vi "ClimbLogic.vi"(0 "FrontClimbEncoder":dbl, 5 "BackClimbEncoder":dbl) -> (4 "ClimbDrive":dbl, 6 "ActuateFrontClimb":dbl, 8 "ActuateBackClimb":dbl)   [LabVIEW 2018]
uses:
  <vilib>/Rock Robotics/WPI/Utilities/WPI_GetSetVariantRefNum.vi
  Swerve/SwerveGlobals.vi
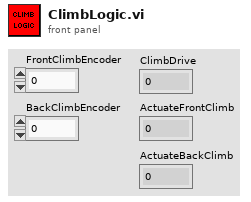
[diagram p1: front panel]
types:
  T1 = typedef "WPI_CompressorDevRef.ctl" = cluster{"DevStatus":errorcluster, "Pneumatics Control Module":u8}
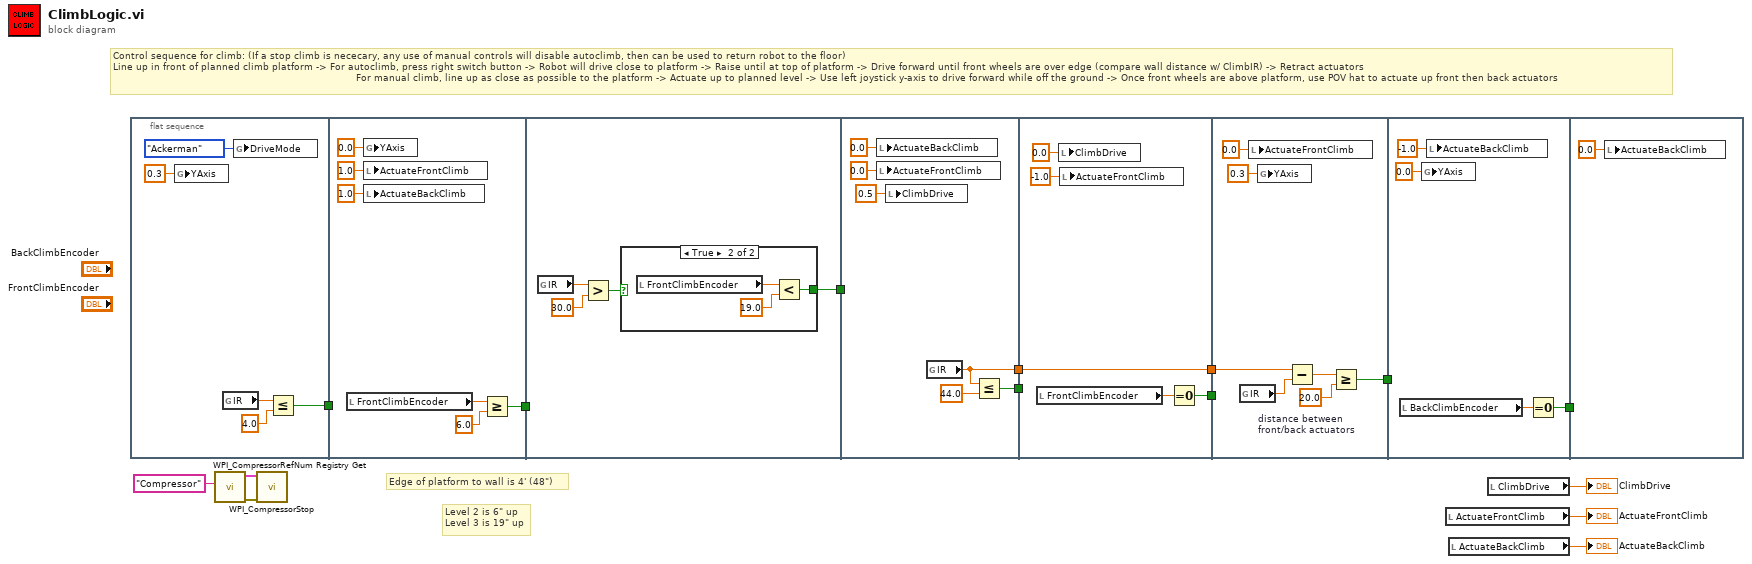
[diagram p0: block diagram]
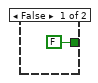
[diagram p2: hidden frame]
diagram:
  # "Level 2 is 6\" up\nLevel 3 is 19\" up"
  # "Edge of platform to wall is 4' (48\")"
  # "Control sequence for climb: (If a stop climb is nececary, any use of manual controls will disable autoclimb, then can be used to return robot to the floor)\nLine up in front of planned climb platform -> For autoclimb, press right switch button -> Robot will drive close to platform -> Raise until at top of platform -> Drive forward until front wheels are over edge (compare wall distance w/ ClimbIR) -> Retract actuators\n                                                                                 For manual climb, line up as close as possible to the platform -> Actuate up to planned level -> Use left joystick y-axis to drive forward while off the ground -> Once front wheels are above platform, use POV hat to actuate up front then back actuators"
  n1 = flat-sequence {
    tunnel: [w17] -> w12
    tunnel: w12 -> [_]
    tunnel: [w21] -> w11
    tunnel: w11 -> [_]
    tunnel: [w27] -> w10
    tunnel: w10 -> [_]
    tunnel: [w36] -> w5
    tunnel: [w35] -> w3
    tunnel: w5 -> [_]
    tunnel: [w43] -> w4
    tunnel: w3 -> [w43]
    tunnel: [w41] -> w2
    tunnel: [w48] -> w9
    tunnel: w4 -> [w47]
    tunnel: w2 -> [_]
    tunnel: w9 -> [_]
    tunnel: [w53] -> w1
    tunnel: w1 -> [_]
    frame #0 {
      n2 = global write "SwerveGlobals.vi" "YAxis"(0.3 ("YAxis")) -> ()
      n3 = global read "SwerveGlobals.vi" "IR"() -> (w16:dbl)
      n4 = global write "SwerveGlobals.vi" "DriveMode"(enum16{"Swerve", "Ackerman"}."Ackerman" ("DriveMode")) -> ()
      n5 = Less Or Equal?(x=w16, y=4.0) -> (x <= y?=w17:bool)
    }
    frame #1 {
      n6 = local read "FrontClimbEncoder"() -> (w23:dbl)
      n7 = global write "SwerveGlobals.vi" "YAxis"(0.0 ("YAxis")) -> ()
      n8 = local write "ActuateFrontClimb"(1.0 ("ActuateFrontClimb")) -> ()
      n9 = local write "ActuateBackClimb"(1.0 ("ActuateBackClimb")) -> ()
      n10 = Greater Or Equal?(x=w23, y=6.0) -> (x >= y?=w21:bool)
    }
    frame #2 {
      n11 = global read "SwerveGlobals.vi" "IR"() -> (w29:dbl)
      n12 = Greater?(x=w29, y=30.0) -> (0:w30:bool)
      n13 = case shown="True" w30 {
        tunnel: [FALSE w32] -> w27
        frame False {
        }
        frame True {
          n14 = local read "FrontClimbEncoder"() -> (w33:dbl)
          n15 = Less?(x=w33, y=19.0) -> (x < y?=w32:bool)
        }
      }
    }
    frame #3 {
      n16 = local write "ActuateBackClimb"(0.0 ("ActuateBackClimb")) -> ()
      n17 = local write "ActuateFrontClimb"(0.0 ("ActuateFrontClimb")) -> ()
      n18 = local write "ClimbDrive"(0.5 ("ClimbDrive")) -> ()
      n19 = global read "SwerveGlobals.vi" "IR"() -> (w35:dbl)
      n20 = Less Or Equal?(x=w35, y=44.0) -> (x <= y?=w36:bool)
    }
    frame #4 {
      n21 = local read "FrontClimbEncoder"() -> (w42:dbl)
      n22 = local write "ClimbDrive"(0.0 ("ClimbDrive")) -> ()
      n23 = local write "ActuateFrontClimb"(-1.0 ("ActuateFrontClimb")) -> ()
      n24 = Equal To 0?(x=w42) -> (x = 0?=w41:bool)
    }
    frame #5 {
      w50 = 20.0  # distance between front/back actuators
      n25 = global read "SwerveGlobals.vi" "IR"() -> (w46:dbl)
      n26 = local write "ActuateFrontClimb"(0.0 ("ActuateFrontClimb")) -> ()
      n27 = global write "SwerveGlobals.vi" "YAxis"(0.3 ("YAxis")) -> ()
      n28 = Subtract(x=w47, y=w46) -> (x-y=w49:dbl)
      n29 = Greater Or Equal?(x=w49, y=w50) -> (x >= y?=w48:bool)
    }
    frame #6 {
      n30 = local read "BackClimbEncoder"() -> (w54:dbl)
      n31 = global write "SwerveGlobals.vi" "YAxis"(0.0 ("YAxis")) -> ()
      n32 = local write "ActuateBackClimb"(-1.0 ("ActuateBackClimb")) -> ()
      n33 = Equal To 0?(x=w54) -> (x = 0?=w53:bool)
    }
    frame #7 {
      n34 = local write "ActuateBackClimb"(0.0 ("ActuateBackClimb")) -> ()
    }
  }
  n35 = call <vilib>:"WPI_CompressorRefNum Registry Get.vi"("refnum name"="Compressor") -> ("error out"=w7:errorcluster, "CompressorDevRef"=w8:T1)  [unwired: 9 in]
  n36 = call <vilib>:"WPI_CompressorStop.vi"("error in (no error)"=w7, "CompressorDevRef"=w8) -> ()  [unwired: 8 in, 2 out]
  n37 = local read "ActuateFrontClimb"() -> (→"ActuateFrontClimb":dbl)
  n38 = local read "ActuateBackClimb"() -> (→"ActuateBackClimb":dbl)
  n39 = local read "ClimbDrive"() -> (→"ClimbDrive":dbl)
